vi "indexFormatCopyFromTreeToTable.vi"(6 "rowNum":u32, 8 "error in":errorcluster, 9 "searchItem":string, 10 "Tree Refnum In":refnum<vi>, 11 "Tbl Refnum in":refnum<vi>) -> (0 "error out":errorcluster, 2 "Tree Refnum Out":refnum<vi>, 3 "Tbl Refnum Out":refnum<vi>)   [LabVIEW 2010]
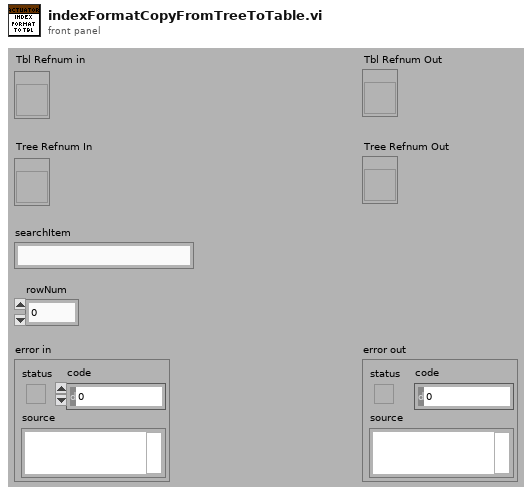
[diagram p1: front panel]
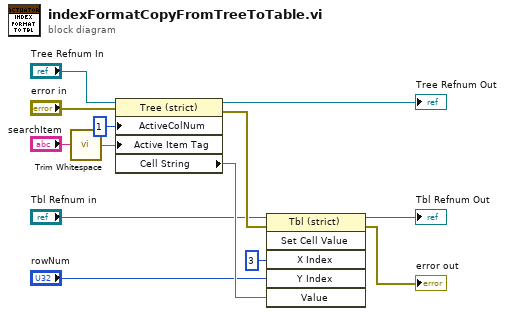
[diagram p0: block diagram]
diagram:
  n1 = call <vilib>:"Trim Whitespace.vi"("string"="searchItem") -> ("trimmed string"=w1:string)  [unwired: 1 in]
  n2 = property class="Tree (strict)"(reference="Tree Refnum In", error in="error in", "ActiveColNum"=1 ("Active Cell:Active Column Number"), "Active Item Tag"=w1) -> (reference out=→"Tree Refnum Out":refnum<vi>, error out=w11:errorcluster, "Cell String"=w10:string)
  n3 = invoke class="Tbl (strict)" method="Set Cell Value"(reference="Tbl Refnum in", error in=w11, "X Index"=u32 3, "Y Index"="rowNum", "Value"=w10) -> (reference out=→"Tbl Refnum Out":refnum<vi>, error out=→"error out":errorcluster)  [unwired: 1 in, 4 out]
